vi "COPY_TEST_Approach-Retraction-VI-NanoHS50-Host-with-averager-2013-04-23-1a-data-storage-no-real-time-display.vi"() -> ()   [LabVIEW 2012]
uses:
  <vilib>/rvi/interface/nirviOpenFPGA/nirviOpenFPGA.xnode
  <vilib>/rvi/interface/nirviReadWriteControl/nirviReadWriteControl.xnode
  <vilib>/rvi/interface/nirviCloseFPGA/nirviCloseFPGA.xnode
  <vilib>/rvi/interface/nirviMethod/nirviMethod.xnode
  <vilib>/rvi/errors/niLvFpgaMergeErrorWithErrorCode.vi
  <vilib>/Utility/file.llb/Write To Spreadsheet File (I64).vi
  <vilib>/FPGAPlugInAG/PCI-7831R/niLvFpga_Open_PCI-7831R.vi
  NiFpgaLv.dll
  <vilib>/Utility/error.llb/Error Cluster From Error Code.vi
  <vilib>/rvi/errors/niLvFpgaAdjustHostInterfaceError.vi
  <vilib>/FPGAPlugInAG/PCI-7831R/niLvFpga_ReadFifo_PCI-7831R.vi
  <vilib>/FPGAPlugInAG/PCI-7831R/niLvFpga_Close_PCI-7831R.vi
  Documents/FPGA-project-apporach-retraction/FPGA Bitfiles/Apporach-Retract_FPGATarget_Automatic-Approa_WyO6UgcJbxk.lvbitx
  Downloads/labview/Automatic-Approach-Retraction-MCL-2013-04-28-1a-data-storage-1b.vi
  <vilib>/FPGAPlugInAG/PCI-7831R/niLvFpga_Run_PCI-7831R.vi
  <vilib>/FPGAPlugInAG/PCI-7831R/niLvFpga_Abort_PCI-7831R.vi
panel:
  out "Base-file-name":string="approach-15a1"
  out "Final file name":path=path "C:/Users/Rodolfo/Documents/LAB/2013-05-16-SPM-data/approach-15a1.txt"
  in  "Data Acquisition\nRate (usec)":u32=2000
  in  "start acquisition - non curve":bool
  in  "base path":path=path "C:/Users/Rodolfo/Documents/LAB/2013-05-16-SPM-data"
  in  "name-file":string="approach-15a"
  out "Data storage":bool
  in  "10 nm step":i16
  in  "variable steps":bool
  out "x*y 2":dbl=125.0
  out "x*y":dbl=3333.3333333333276
  in  "Safetip Control ON/Off":bool
  in  "safetip time wait":u32=65534
  in  "Safetip retraction":u16=1
  out "AI2-data2file":i16[](array[numeric])=[-198, -198, -198, -198, -198, -198, -198, -198, -198, -198, -197, -197, -197, -197, -197, -197, -197, -197, -197, -197, -197, -197, -197, -197, -197, -197, -196, -197, -196, -196, -196, -196, -196, -196, -196, -196, -196, -196, -196, -196, -196, -196, -196, -196, -196, -196, -196, -195, -195, -195, -195, -195, -195, -195, -195, -195, -195, -195, -195, -195, -195, -195, -195, -195, -195, -194, -194, -194, -194, -194, -194, -194, -194, -194, -194, -194, -194, -194, -194, -194, -194, -194, -194, -193, -193, -193, -193, -193, -193, -193, -193, -193, -193, -193, -193, -193, -193, -193, -193, -193, -193, -193, -193, -193, -193, -192, -192, -192, -192, -192, -192, -192, -192, -192, -192, -192, -192, -192, -192, -192, -192, -192, -191, -191, -191, -191, -191, -191, -191, -191, -191, -191, -191, -191, -191, -191, -191, -191, -191, -191, -191, -191, -190, -190, -190, -190, -190, -190, -190, -190, -190, -190, -190, -190, -190, -190, -190, -190, -190, -190, -189, -189, -189, -189, -189, -189, -189, -189, -189, -189, -189, -189, -189, -189, -189, -189, -189, -189, -188, -188, -188, -188, -188, -188, -188, -188, -188, -188, -188, -188, -188, -188, -188, -188, -188, -188, -188, -188, -187, -188, -187, -187, -187, -187, -187, -187, -187, -187, -187, -187, -187, -187, -187, -187, -187, -187, -186, -186, -186, -186, -186, -186, -186, -186, -186, -186, -186, -186, -186, -186, -186, -186, -186, -186, -186, -186, -186, -185, -185, -185, -185, -185, -185, -185, -185, -185, -185, -185, -185, -185, -185, -185, -185, -185, -185, -184, -184, -184, -184, -184, -184, -184, -184, -184, -184, -184, -184, -184, -184, -184, -184, -184, -184, -183, -184, -183, -183, -183, -183, -183, -183, -183, -183, -183, -183, -183, -183, -183, -183, -183, -183, -182, -182, -182, -182, -182, -182, -182, -182, -182, -182, -182, -182, -182, -182, -182, -182, -182, -182, -182, -182, -182, -181, -181, -181, -181, -181, -181, -181, -181, -181, -181, -181, -181, -181, -181, -181, -181, -181, -180, -180, -180, -180, -180, -180, -180, -180, -180, -180, -180, -180, -180, -180, -180, -180, -180, -180, -180, -179, -179, -180, -179, -179, -179, -179, -179, -179, -179, -179, -179, -179, -179, -179, -179, -179, -179, -179, -178, -178, -178, -178, -178, -178, -178, -178, -178, -178, -178, -178, -178, -178, -178, -178, -178, -178, -178, -177, -178, -177, -177, -177, -177, -177, -177, -177, -177, -177, -177, -177, -177, -177, -177, -177, -177, -177, -177, -176, -176, -176, -176, -176, -176, -176, -176, -176, -176, -176, -176, -176, -176, -176, -176, -175, -175, -175, -175, -175, -175, -175, -175, -175, -175, -175, -175, -175, -175, -175, -175, -175, -175, -175, -175, -175, -175, -174, -174, -174, -174, -174, -174, -174, -174, -174, -174, -174, -174, -174, -174, -174, -174, -174, -173, -174, -173, -173, -173, -173, -173, -173, -173, -173, -173, -173, -173, -173, -173, -173, -173, -173, -173, -173, -172, -172, -172, -172, -172, -172, -172, -172, -172, -172, -172, -172, -172, -172, -172, -172, -172, -171, -171]
  out "AI5-data2file":i16[](array[numeric])=[286, 288, 287, 294, 295, 295, 294, 294, 301, 300, 301, 299, 299, 297, 297, 297, 297, 297, 304, 304, 305, 307, 307, 306, 306, 308, 315, 314, 310, 311, 310, 310, 310, 310, 310, 310, 309, 309, 311, 311, 309, 307, 307, 304, 304, 301, 297, 297, 286, 286, 284, 281, 282, 271, 272, 267, 260, 260, 251, 251, 248, 244, 244, 238, 238, 235, 231, 232, 226, 226, 221, 214, 215, 201, 202, 197, 192, 192, 181, 183, 181, 180, 180, 169, 170, 169, 168, 168, 163, 163, 164, 167, 167, 167, 167, 167, 167, 167, 168, 168, 168, 169, 169, 172, 172, 176, 180, 180, 190, 189, 192, 195, 195, 210, 208, 214, 219, 218, 233, 231, 238, 242, 242, 254, 253, 262, 269, 268, 278, 277, 283, 288, 288, 302, 300, 308, 313, 313, 325, 323, 327, 329, 329, 338, 336, 343, 347, 347, 356, 354, 360, 362, 362, 365, 365, 365, 366, 366, 366, 366, 363, 361, 360, 352, 353, 350, 349, 349, 340, 341, 335, 333, 332, 321, 322, 321, 320, 320, 316, 316, 315, 314, 314, 310, 311, 305, 303, 303, 300, 301, 300, 299, 299, 297, 297, 292, 291, 290, 282, 282, 279, 278, 277, 273, 273, 274, 274, 274, 274, 274, 273, 273, 273, 274, 274, 276, 276, 277, 282, 281, 284, 284, 284, 286, 286, 287, 287, 287, 286, 286, 284, 284, 284, 281, 282, 278, 277, 276, 271, 272, 267, 267, 266, 264, 264, 261, 261, 260, 256, 257, 258, 258, 257, 253, 253, 249, 249, 247, 241, 242, 232, 231, 229, 221, 222, 212, 211, 210, 205, 205, 200, 199, 198, 190, 191, 183, 183, 182, 178, 179, 180, 180, 180, 180, 180, 182, 181, 181, 180, 180, 184, 185, 186, 190, 190, 190, 190, 190, 191, 191, 190, 190, 190, 191, 190, 195, 196, 199, 210, 209, 221, 221, 225, 237, 235, 247, 247, 251, 262, 261, 272, 271, 275, 280, 280, 294, 294, 296, 299, 299, 307, 307, 309, 315, 314, 319, 319, 320, 324, 324, 328, 328, 331, 337, 337, 343, 343, 345, 349, 349, 360, 360, 362, 365, 364, 370, 369, 369, 369, 369, 365, 365, 365, 366, 366, 361, 361, 361, 360, 360, 360, 360, 360, 358, 358, 360, 360, 359, 358, 359, 356, 356, 353, 350, 350, 346, 345, 346, 347, 347, 341, 342, 341, 340, 340, 333, 333, 333, 331, 332, 327, 327, 325, 322, 322, 320, 320, 320, 320, 320, 317, 317, 318, 320, 320, 318, 319, 321, 324, 324, 324, 324, 326, 326, 326, 330, 329, 333, 336, 336, 348, 346, 352, 357, 356, 362, 361, 364, 366, 366, 368, 368, 371, 373, 373, 373, 373, 371, 368, 368, 370, 369, 371, 372, 372, 373, 373, 373, 373, 373, 375, 374, 375, 375, 375, 367, 368, 366, 366, 365, 359, 360, 357, 355, 355, 350, 350, 344, 342, 341, 336, 337, 330, 327, 326, 319, 319, 313, 310, 310, 305, 305, 302, 301, 300, 297, 297, 297, 296, 296]
  out "Top-data2file":i32[](array[numeric])=[6625035, 6625035, 6625035, 6625035, 6625035, 6625035, 6625035, 6625035, 6625035, 6625035, 6625035, 6625035, 6625035, 6625035, 6625035, 6625035, 6625035, 6625035, 6625035, 6625035, 6625035, 6625035, 6625035, 6625035, 6625035, 6625035, 6625035, 6625035, 6625035, 6625035, 6625035, 6625035, 6625035, 6625035, 6625035, 6625035, 6625035, 6625035, 6625035, 6625035, 6625035, 6625035, 6625035, 6625035, 6625035, 6625035, 6625035, 6625035, 6625035, 6625035, 6625035, 6625035, 6625035, 6625035, 6625035, 6625035, 6625035, 6625035, 6625035, 6625035, 6625035, 6625035, 6625035, 6625035, 6625035, 6625035, 6625035, 6625035, 6625035, 6625035, 6625035, 6625035, 6625035, 6625035, 6625035, 6625035, 6625035, 6625035, 6625035, 6625035, 6625035, 6625035, 6625035, 6625035, 6625035, 6625035, 6625035, 6625035, 6625035, 6625035, 6625035, 6625035, 6625035, 6625035, 6625035, 6625035, 6625035, 6625035, 6625035, 6625035, 6625035, 6625035, 6625035, 6625035, 6625035, 6625035, 6625035, 6625035, 6625035, 6625035, 6625035, 6625035, 6625035, 6625035, 6625035, 6625035, 6625035, 6625035, 6625035, 6625035, 6625035, 6625035, 6625035, 6625035, 6625035, 6625035, 6625035, 6625035, 6625035, 6625035, 6625035, 6625035, 6625035, 6625035, 6625035, 6625035, 6625035, 6625035, 6625035, 6625035, 6625035, 6625035, 6625035, 6625035, 6625035, 6625035, 6625035, 6625035, 6625035, 6625035, 6625035, 6625035, 6625035, 6625035, 6625035, 6625035, 6625035, 6625035, 6625035, 6625035, 6625035, 6625035, 6625035, 6625035, 6625035, 6625035, 6625035, 6625035, 6625035, 6625035, 6625035, 6625035, 6625035, 6625035, 6625035, 6625035, 6625035, 6625035, 6625035, 6625035, 6625035, 6625035, 6625035, 6625035, 6625035, 6625035, 6625035, 6625035, 6625035, 6625035, 6625035, 6625035, 6625035, 6625035, 6625035, 6625035, 6625035, 6625035, 6625035, 6625035, 6625035, 6625035, 6625035, 6625035, 6625035, 6625035, 6625035, 6625035, 6625035, 6625035, 6625035, 6625035, 6625035, 6625035, 6625035, 6625035, 6625035, 6625035, 6625035, 6625035, 6625035, 6625035, 6625035, 6625035, 6625035, 6625035, 6625035, 6625035, 6625035, 6625035, 6625035, 6625035, 6625035, 6625035, 6625035, 6625035, 6625035, 6625035, 6625035, 6625035, 6625035, 6625035, 6625035, 6625035, 6625035, 6625035, 6625035, 6625035, 6625035, 6625035, 6625035, 6625035, 6625035, 6625035, 6625035, 6625035, 6625035, 6625035, 6625035, 6625035, 6625035, 6625035, 6625035, 6625035, 6625035, 6625035, 6625035, 6625035, 6625035, 6625035, 6625035, 6625035, 6625035, 6625035, 6625035, 6625035, 6625035, 6625035, 6625035, 6625035, 6625035, 6625035, 6625035, 6625035, 6625035, 6625035, 6625035, 6625035, 6625035, 6625035, 6625035, 6625035, 6625035, 6625035, 6625035, 6625035, 6625035, 6625035, 6625035, 6625035, 6625035, 6625035, 6625035, 6625035, 6625035, 6625035, 6625035, 6625035, 6625035, 6625035, 6625035, 6625035, 6625035, 6625035, 6625035, 6625035, 6625035, 6625035, 6625035, 6625035, 6625035, 6625035, 6625035, 6625035, 6625035, 6625035, 6625035, 6625035, 6625035, 6625035, 6625035, 6625035, 6625035, 6625035, 6625035, 6625035, 6625035, 6625035, 6625035, 6625035, 6625035, 6625035, 6625035, 6625035, 6625035, 6625035, 6625035, 6625035, 6625035, 6625035, 6625035, 6625035, 6625035, 6625035, 6625035, 6625035, 6625035, 6625035, 6625035, 6625035, 6625035, 6625035, 6625035, 6625035, 6625035, 6625035, 6625035, 6625035, 6625035, 6625035, 6625035, 6625035, 6625035, 6625035, 6625035, 6625035, 6625035, 6625035, 6625035, 6625035, 6625035, 6625035, 6625035, 6625035, 6625035, 6625035, 6625035, 6625035, 6625035, 6625035, 6625035, 6625035, 6625035, 6625035, 6625035, 6625035, 6625035, 6625035, 6625035, 6625035, 6625035, 6625035, 6625035, 6625035, 6625035, 6625035, 6625035, 6625035, 6625035, 6625035, 6625035, 6625035, 6625035, 6625035, 6625035, 6625035, 6625035, 6625035, 6625035, 6625035, 6625035, 6625035, 6625035, 6625035, 6625035, 6625035, 6625035, 6625035, 6625035, 6625035, 6625035, 6625035, 6625035, 6625035, 6625035, 6625035, 6625035, 6625035, 6625035, 6625035, 6625035, 6625035, 6625035, 6625035, 6625035, 6625035, 6625035, 6625035, 6625035, 6625035, 6625035, 6625035, 6625035, 6625035, 6625035, 6625035, 6625035, 6625035, 6625035, 6625035, 6625035, 6625035, 6625035, 6625035, 6625035, 6625035, 6625035, 6625035, 6625035, 6625035, 6625035, 6625035, 6625035, 6625035, 6625035, 6625035, 6625035, 6625035, 6625035, 6625035, 6625035, 6625035, 6625035, 6625035, 6625035, 6625035, 6625035, 6625035, 6625035, 6625035, 6625035, 6625035, 6625035, 6625035, 6625035, 6625035, 6625035, 6625035, 6625035, 6625035]
  out "AI6-data2file":i16[](array[numeric])=[10327, 10323, 10323, 10324, 10324, 10324, 10323, 10323, 10321, 10320, 10320, 10318, 10318, 10312, 10310, 10309, 10304, 10305, 10298, 10296, 10296, 10301, 10301, 10298, 10297, 10297, 10290, 10290, 10294, 10295, 10295, 10296, 10296, 10303, 10304, 10305, 10309, 10308, 10308, 10307, 10307, 10309, 10308, 10309, 10309, 10310, 10319, 10318, 10318, 10318, 10318, 10317, 10317, 10310, 10308, 10308, 10307, 10307, 10308, 10308, 10308, 10304, 10304, 10298, 10296, 10295, 10291, 10291, 10287, 10286, 10286, 10285, 10285, 10290, 10291, 10292, 10294, 10294, 10295, 10295, 10295, 10294, 10294, 10297, 10297, 10298, 10301, 10301, 10307, 10307, 10308, 10311, 10311, 10310, 10309, 10311, 10319, 10318, 10320, 10320, 10320, 10319, 10319, 10320, 10320, 10320, 10319, 10319, 10318, 10318, 10317, 10314, 10314, 10308, 10307, 10307, 10304, 10304, 10307, 10307, 10307, 10308, 10308, 10310, 10311, 10312, 10314, 10314, 10314, 10314, 10315, 10317, 10317, 10318, 10318, 10318, 10318, 10318, 10314, 10313, 10313, 10311, 10311, 10307, 10307, 10307, 10309, 10308, 10308, 10308, 10308, 10308, 10308, 10308, 10308, 10307, 10303, 10303, 10301, 10301, 10301, 10301, 10301, 10304, 10303, 10305, 10309, 10308, 10310, 10309, 10313, 10321, 10320, 10324, 10324, 10329, 10337, 10336, 10341, 10341, 10341, 10342, 10342, 10341, 10341, 10337, 10331, 10331, 10317, 10317, 10314, 10310, 10311, 10303, 10303, 10300, 10294, 10295, 10287, 10288, 10288, 10287, 10287, 10285, 10285, 10286, 10286, 10286, 10295, 10295, 10297, 10301, 10301, 10311, 10310, 10314, 10318, 10318, 10319, 10319, 10323, 10328, 10328, 10334, 10333, 10335, 10337, 10337, 10337, 10337, 10337, 10336, 10336, 10331, 10331, 10329, 10327, 10327, 10324, 10324, 10322, 10320, 10320, 10313, 10313, 10314, 10314, 10314, 10308, 10308, 10306, 10304, 10304, 10309, 10308, 10303, 10299, 10300, 10301, 10301, 10302, 10305, 10304, 10300, 10301, 10303, 10305, 10304, 10303, 10303, 10304, 10305, 10305, 10308, 10308, 10308, 10308, 10308, 10315, 10314, 10316, 10317, 10317, 10321, 10320, 10324, 10328, 10328, 10334, 10333, 10336, 10337, 10337, 10340, 10339, 10342, 10343, 10343, 10343, 10343, 10346, 10347, 10347, 10347, 10347, 10349, 10349, 10349, 10347, 10347, 10344, 10343, 10343, 10343, 10343, 10343, 10343, 10343, 10339, 10340, 10338, 10337, 10337, 10333, 10334, 10327, 10324, 10324, 10320, 10320, 10318, 10317, 10316, 10310, 10311, 10300, 10297, 10296, 10284, 10286, 10285, 10285, 10285, 10284, 10284, 10287, 10288, 10289, 10298, 10297, 10303, 10304, 10306, 10319, 10317, 10330, 10332, 10334, 10348, 10347, 10349, 10350, 10350, 10355, 10354, 10354, 10354, 10354, 10349, 10349, 10344, 10343, 10342, 10332, 10334, 10326, 10324, 10323, 10313, 10315, 10310, 10310, 10309, 10308, 10308, 10304, 10304, 10302, 10294, 10295, 10292, 10291, 10290, 10286, 10287, 10285, 10285, 10285, 10281, 10281, 10285, 10285, 10286, 10288, 10288, 10290, 10290, 10291, 10295, 10295, 10299, 10300, 10302, 10312, 10311, 10320, 10320, 10321, 10323, 10323, 10320, 10320, 10321, 10324, 10323, 10324, 10324, 10325, 10328, 10327, 10327, 10326, 10328, 10332, 10331, 10330, 10330, 10332, 10338, 10337, 10341, 10341, 10340, 10336, 10336, 10334, 10333, 10333, 10330, 10331, 10331, 10331, 10330, 10327, 10328, 10330, 10330, 10328, 10323, 10324, 10317, 10317, 10316, 10314, 10315, 10314, 10314, 10312, 10307, 10307, 10301, 10301, 10297, 10290, 10291, 10285, 10285, 10283, 10277, 10278, 10277, 10277, 10279, 10282, 10282, 10286, 10286, 10288, 10292, 10291, 10301, 10300, 10304, 10308, 10307, 10318, 10318, 10320, 10324, 10323]
  out "AI1-data2file":i16[](array[numeric])
  out "AI7-data2file":i16[](array[numeric])=[26628, 26626, 26633, 26632, 26632, 26626, 26648, 26626, 26639, 26625, 26644, 26635, 26624, 26639, 26643, 26622, 26621, 26637, 26626, 26627, 26641, 26632, 26634, 26652, 26632, 26635, 26620, 26631, 26645, 26637, 26634, 26631, 26640, 26634, 26640, 26632, 26637, 26642, 26623, 26629, 26624, 26638, 26636, 26646, 26622, 26644, 26622, 26624, 26636, 26632, 26636, 26617, 26628, 26639, 26639, 26626, 26628, 26650, 26634, 26626, 26641, 26620, 26628, 26639, 26625, 26646, 26618, 26649, 26627, 26641, 26625, 26638, 26636, 26636, 26638, 26639, 26638, 26640, 26642, 26641, 26639, 26628, 26638, 26629, 26639, 26631, 26638, 26638, 26625, 26636, 26635, 26628, 26652, 26635, 26632, 26628, 26644, 26632, 26644, 26638, 26633, 26616, 26630, 26629, 26623, 26630, 26623, 26633, 26626, 26644, 26636, 26643, 26625, 26632, 26632, 26633, 26630, 26623, 26623, 26636, 26632, 26631, 26637, 26632, 26633, 26640, 26646, 26632, 26635, 26629, 26635, 26621, 26633, 26634, 26628, 26642, 26634, 26629, 26619, 26639, 26632, 26632, 26636, 26634, 26637, 26633, 26644, 26631, 26647, 26626, 26646, 26628, 26633, 26642, 26653, 26640, 26633, 26638, 26633, 26620, 26641, 26640, 26630, 26621, 26621, 26644, 26642, 26634, 26641, 26627, 26615, 26640, 26633, 26639, 26628, 26634, 26647, 26623, 26625, 26635, 26639, 26640, 26629, 26640, 26614, 26656, 26630, 26649, 26652, 26630, 26637, 26620, 26638, 26632, 26638, 26646, 26633, 26628, 26645, 26636, 26639, 26632, 26633, 26649, 26627, 26633, 26629, 26631, 26629, 26643, 26627, 26631, 26637, 26635, 26648, 26629, 26635, 26636, 26640, 26627, 26640, 26608, 26640, 26629, 26632, 26646, 26632, 26629, 26631, 26621, 26643, 26640, 26618, 26623, 26640, 26640, 26639, 26628, 26630, 26636, 26631, 26642, 26633, 26639, 26633, 26647, 26624, 26630, 26631, 26646, 26630, 26636, 26638, 26636, 26647, 26638, 26625, 26625, 26631, 26625, 26639, 26638, 26641, 26625, 26650, 26634, 26643, 26607, 26660, 26623, 26642, 26649, 26631, 26633, 26632, 26641, 26627, 26632, 26641, 26627, 26646, 26629, 26618, 26635, 26630, 26643, 26627, 26639, 26630, 26625, 26625, 26639, 26641, 26626, 26638, 26630, 26628, 26649, 26637, 26632, 26625, 26630, 26641, 26638, 26636, 26632, 26627, 26628, 26629, 26642, 26631, 26619, 26636, 26628, 26631, 26634, 26633, 26640, 26627, 26645, 26628, 26633, 26625, 26637, 26617, 26628, 26637, 26642, 26628, 26643, 26637, 26637, 26629, 26632, 26629, 26633, 26626, 26637, 26630, 26635, 26637, 26653, 26634, 26636, 26638, 26623, 26629, 26638, 26630, 26638, 26649, 26622, 26640, 26635, 26629, 26627, 26651, 26643, 26652, 26625, 26631, 26627, 26637, 26631, 26626, 26630, 26627, 26646, 26629, 26644, 26632, 26652, 26636, 26628, 26644, 26651, 26623, 26639, 26622, 26643, 26635, 26661, 26635, 26630, 26631, 26638, 26631, 26632, 26629, 26625, 26629, 26627, 26622, 26636, 26637, 26628, 26638, 26631, 26625, 26627, 26630, 26639, 26646, 26629, 26631, 26650, 26620, 26634, 26634, 26652, 26626, 26644, 26639, 26639, 26646, 26646, 26631, 26640, 26630, 26638, 26638, 26651, 26633, 26631, 26622, 26641, 26639, 26639, 26637, 26633, 26630, 26647, 26619, 26640, 26641, 26630, 26642, 26633, 26629, 26641, 26623, 26631, 26647, 26618, 26641, 26630, 26638, 26631, 26634, 26631, 26633, 26637, 26631, 26635, 26635, 26637, 26640, 26636, 26631, 26634, 26644, 26632, 26642, 26630, 26626, 26629, 26641, 26641, 26636, 26640, 26639, 26639, 26629, 26640, 26629, 26647, 26625, 26647, 26651, 26636, 26633, 26625, 26629, 26638, 26644, 26639, 26602, 26636, 26621, 26629, 26636, 26643, 26633, 26640, 26632, 26631, 26633, 26636, 26624, 26627]
  out "AI4-data2file":i16[](array[numeric])=[355, 354, 354, 355, 355, 354, 353, 352, 351, 350, 351, 351, 350, 349, 350, 350, 350, 351, 352, 353, 353, 353, 352, 350, 349, 346, 345, 345, 342, 340, 339, 341, 342, 342, 344, 345, 345, 346, 348, 348, 347, 348, 348, 347, 346, 346, 345, 346, 344, 345, 347, 348, 349, 350, 350, 352, 353, 353, 353, 352, 351, 350, 350, 352, 353, 353, 355, 354, 353, 353, 355, 353, 355, 354, 355, 356, 356, 356, 354, 352, 352, 350, 350, 350, 350, 350, 350, 350, 350, 348, 347, 345, 346, 346, 346, 346, 346, 346, 345, 344, 346, 346, 347, 347, 349, 349, 347, 347, 346, 348, 349, 349, 349, 349, 349, 349, 349, 348, 351, 350, 350, 352, 354, 355, 354, 353, 351, 350, 349, 347, 348, 347, 347, 345, 345, 345, 345, 345, 345, 345, 347, 346, 346, 345, 345, 344, 346, 346, 346, 347, 348, 351, 350, 350, 350, 350, 352, 352, 352, 350, 350, 350, 350, 350, 350, 351, 351, 350, 350, 349, 348, 347, 345, 345, 347, 349, 349, 349, 349, 349, 350, 350, 352, 352, 351, 349, 346, 346, 345, 343, 342, 340, 341, 341, 341, 340, 340, 341, 340, 340, 341, 343, 345, 345, 348, 349, 349, 350, 350, 351, 351, 350, 350, 350, 351, 351, 351, 350, 350, 352, 353, 353, 353, 355, 355, 355, 355, 355, 353, 352, 352, 352, 352, 353, 353, 355, 355, 354, 355, 355, 355, 355, 355, 353, 353, 351, 350, 350, 350, 350, 351, 350, 350, 350, 350, 350, 351, 351, 352, 353, 353, 353, 353, 353, 355, 356, 356, 357, 359, 359, 359, 359, 359, 359, 359, 359, 359, 358, 359, 359, 359, 359, 359, 359, 357, 358, 357, 356, 354, 353, 352, 351, 350, 349, 349, 348, 347, 347, 345, 344, 345, 345, 345, 344, 345, 346, 347, 348, 351, 350, 350, 353, 353, 353, 353, 353, 352, 350, 351, 350, 347, 346, 345, 346, 346, 346, 347, 349, 350, 352, 353, 352, 351, 351, 351, 351, 350, 350, 350, 349, 349, 349, 349, 348, 348, 346, 346, 346, 346, 346, 349, 349, 351, 350, 350, 352, 355, 354, 355, 355, 354, 351, 350, 350, 351, 352, 352, 354, 355, 355, 354, 353, 352, 350, 350, 350, 348, 347, 345, 344, 344, 343, 344, 342, 342, 342, 343, 344, 345, 349, 350, 352, 355, 356, 356, 356, 356, 355, 354, 352, 353, 350, 351, 350, 350, 349, 349, 349, 349, 348, 346, 346, 346, 345, 345, 345, 344, 343, 343, 344, 345, 344, 345, 344, 345, 345, 345, 345, 345, 343, 342, 342, 340, 342, 340, 341, 341, 343, 343, 345, 344, 345, 345, 345, 345, 344, 345, 345, 345, 345, 347, 348, 348, 349, 349, 349, 348, 347, 346, 345, 345, 344, 343, 343, 342, 342, 343, 343, 345, 345, 345, 345, 346, 347, 349, 349, 351, 350, 350, 350, 350, 350, 350, 349, 349, 349, 348, 347, 346, 345, 345, 346, 347, 347, 346, 345, 345, 345, 345, 345]
  in  "start acquisition":bool
  out "Phase 1":bool
  in  "phase 1 control":bool
  out "Initial Height (Fine)":i16
  out "MCL counter in range?":bool=TRUE
  out "Zposition MCL fine":i16=6000
  out "MCL counter":u16=101
  out "Curve indicator":u16=1
  in  "Manual Control":bool=TRUE
  in  "Start Approach":bool
  in  "Data Length":i32=10000
  in  "MCL  Divisions":u16=102
  in  "MCL counter 2":u16=101
  in  "Zposition MCL fine 2":i16=6000 step=1
  in  "Initial Position":i16
  in  "Safetip Minimum":i16=4700
  in  "Number of curves":u16=5
  in  "Fine Retraction  Velocity (nm/s)":dbl=3.0000000000000053 format="%.2g"
  in  "Wait-tip-before-new-approach (usec)":u32=100000
  in  "Wait-tip-\nbefore-approach (usec)":u32=100001
  in  "Fast Approach\nVelocity (nm/s)":dbl=80.0 min=0.1 max=100.0 step=0.001 format="%_3g"
  in  "Approach Setpoint":i16=16400
  out "Signal away from surface":i16=26655
  in  "First fast\napproach offset":i16=90
  in  "Fast Retraction\nbefore approach":i32=3601 min=0
  in  "Minimum for Approach Value":i16=7800
  in  "Fast Retraction after approach":i32=30000 step=1
  out "AI2":i16[](graph)
  out "AI5":i16[](graph)
  out "Topography":i32[](graph)
  out "AI6":i16[](graph)
  out "AI1":i16[](graph)
  out "AI7":i16[](graph)
  out "AI4":i16[](graph)
  out "Data 2":u64[](array[numeric])=[28454742470360890, 28454742470491962, 28454742470426426, 28454742470885178, 28454742470950714, 28454742470950714, 28454742470885178, 28454742470885178, 28454742471343930, 28454742471278394, 28454742471343931, 28454742471212859, 28454742471212859, 28454742471081787, 28454742471081787, 28454742471081787, 28454742471081787, 28454742471081787, 28454742471540539, 28454742471540539, 28454742471606075, 28454742471737147, 28454742471737147, 28454742471671611, 28454742471671611, 28454742471802683, 28454742472261436, 28454742472195899, 28454742471933756, 28454742471999292, 28454742471933756, 28454742471933756, 28454742471933756, 28454742471933756, 28454742471933756, 28454742471933756, 28454742471868220, 28454742471868220, 28454742471999292, 28454742471999292, 28454742471868220, 28454742471737148, 28454742471737148, 28454742471540540, 28454742471540540, 28454742471343932, 28454742471081788, 28454742471081789, 28454742470360893, 28454742470360893, 28454742470229821, 28454742470033213, 28454742470098749, 28454742469377853, 28454742469443389, 28454742469115709, 28454742468656957, 28454742468656957, 28454742468067133, 28454742468067133, 28454742467870525, 28454742467608381, 28454742467608381, 28454742467215165, 28454742467215165, 28454742467018558, 28454742466756414, 28454742466821950, 28454742466428734, 28454742466428734, 28454742466101054, 28454742465642302, 28454742465707838, 28454742464790334, 28454742464855870, 28454742464528190, 28454742464200510, 28454742464200510, 28454742463479614, 28454742463610686, 28454742463479614, 28454742463414078, 28454742463414078, 28454742462693183, 28454742462758719, 28454742462693183, 28454742462627647, 28454742462627647, 28454742462299967, 28454742462299967, 28454742462365503, 28454742462562111, 28454742462562111, 28454742462562111, 28454742462562111, 28454742462562111, 28454742462562111, 28454742462562111, 28454742462627647, 28454742462627647, 28454742462627647, 28454742462693183, 28454742462693183, 28454742462889791, 28454742462889791, 28454742463151936, 28454742463414080, 28454742463414080, 28454742464069440, 28454742464003904, 28454742464200512, 28454742464397120, 28454742464397120, 28454742465380160, 28454742465249088, 28454742465642304, 28454742465969984, 28454742465904448, 28454742466887488, 28454742466756416, 28454742467215168, 28454742467477312, 28454742467477313, 28454742468263745, 28454742468198209, 28454742468788033, 28454742469246785, 28454742469181249, 28454742469836609, 28454742469771073, 28454742470164289, 28454742470491969, 28454742470491969, 28454742471409473, 28454742471278401, 28454742471802689, 28454742472130369, 28454742472130369, 28454742472916801, 28454742472785729, 28454742473047873, 28454742473178945, 28454742473178946, 28454742473768770, 28454742473637698, 28454742474096450, 28454742474358594, 28454742474358594, 28454742474948418, 28454742474817346, 28454742475210562, 28454742475341634, 28454742475341634, 28454742475538242, 28454742475538242, 28454742475538242, 28454742475603778, 28454742475603778, 28454742475603778, 28454742475603778, 28454742475407171, 28454742475276099, 28454742475210563, 28454742474686275, 28454742474751811, 28454742474555203, 28454742474489667, 28454742474489667, 28454742473899843, 28454742473965379, 28454742473572163, 28454742473441091, 28454742473375555, 28454742472654659, 28454742472720195, 28454742472654659, 28454742472589123, 28454742472589123, 28454742472326980, 28454742472326980, 28454742472261444, 28454742472195908, 28454742472195908, 28454742471933764, 28454742471999300, 28454742471606084, 28454742471475012, 28454742471475012, 28454742471278404, 28454742471343940, 28454742471278404, 28454742471212868, 28454742471212868, 28454742471081796, 28454742471081796, 28454742470754116, 28454742470688580, 28454742470623044, 28454742470098757, 28454742470098756, 28454742469902149, 28454742469836613, 28454742469771077, 28454742469508933, 28454742469508933, 28454742469574469, 28454742469574469, 28454742469574469, 28454742469574469, 28454742469574469, 28454742469508933, 28454742469508933, 28454742469508933, 28454742469574469, 28454742469574469, 28454742469705541, 28454742469705542, 28454742469771078, 28454742470098758, 28454742470033222, 28454742470229830, 28454742470229830, 28454742470229830, 28454742470360902, 28454742470360902, 28454742470426438, 28454742470426438, 28454742470426438, 28454742470360902, 28454742470360902, 28454742470229830, 28454742470229830, 28454742470229830, 28454742470033222, 28454742470098758, 28454742469836614, 28454742469771078, 28454742469705543, 28454742469377863, 28454742469443399, 28454742469115719, 28454742469115719, 28454742469050183, 28454742468919111, 28454742468919111, 28454742468722503, 28454742468722503, 28454742468656967, 28454742468394823, 28454742468460359, 28454742468525895, 28454742468525895, 28454742468460359, 28454742468198215, 28454742468198215, 28454742467936072, 28454742467936072, 28454742467805000, 28454742467411784, 28454742467477320, 28454742466821960, 28454742466756424, 28454742466625352, 28454742466101064, 28454742466166600, 28454742465511240, 28454742465445704, 28454742465380168, 28454742465052488, 28454742465052488, 28454742464724808, 28454742464659272, 28454742464593736, 28454742464069449, 28454742464134984, 28454742463610697, 28454742463610697, 28454742463545161, 28454742463283017, 28454742463348553, 28454742463414089, 28454742463414089, 28454742463414089, 28454742463414089, 28454742463414089, 28454742463545161, 28454742463479625, 28454742463479625, 28454742463414089, 28454742463414089, 28454742463676233, 28454742463741770, 28454742463807306, 28454742464069450, 28454742464069450, 28454742464069450, 28454742464069450, 28454742464069450, 28454742464134986, 28454742464134986, 28454742464069450, 28454742464069450, 28454742464069450, 28454742464134986, 28454742464069450, 28454742464397130, 28454742464462666, 28454742464659274, 28454742465380170, 28454742465314634, 28454742466101066, 28454742466101066, 28454742466363211, 28454742467149643, 28454742467018571, 28454742467805003, 28454742467805003, 28454742468067147, 28454742468788043, 28454742468722507, 28454742469443403, 28454742469377867, 28454742469640011, 28454742469967691, 28454742469967691, 28454742470885195, 28454742470885195, 28454742471016267, 28454742471212875, 28454742471212876, 28454742471737164, 28454742471737164, 28454742471868236, 28454742472261452, 28454742472195916, 28454742472523596, 28454742472523596, 28454742472589132, 28454742472851276, 28454742472851276, 28454742473113420, 28454742473113420, 28454742473310028, 28454742473703244, 28454742473703244, 28454742474096460, 28454742474096460, 28454742474227532, 28454742474489677, 28454742474489677, 28454742475210572, 28454742475210573, 28454742475341645, 28454742475538253, 28454742475472717, 28454742475865933, 28454742475800397, 28454742475800397, 28454742475800397, 28454742475800397, 28454742475538253, 28454742475538253, 28454742475538253, 28454742475603789, 28454742475603789, 28454742475276109, 28454742475276109, 28454742475276110, 28454742475210574, 28454742475210574, 28454742475210574, 28454742475210574, 28454742475210574, 28454742475079502, 28454742475079502, 28454742475210574, 28454742475210574, 28454742475145038, 28454742475079502, 28454742475145038, 28454742474948430, 28454742474948430, 28454742474751822, 28454742474555214, 28454742474555214, 28454742474293070, 28454742474227535, 28454742474293070, 28454742474358607, 28454742474358607, 28454742473965391, 28454742474030927, 28454742473965391, 28454742473899855, 28454742473899855, 28454742473441103, 28454742473441103, 28454742473441103, 28454742473310031, 28454742473375567, 28454742473047887, 28454742473047887, 28454742472916815, 28454742472720207, 28454742472720207, 28454742472589135, 28454742472589136, 28454742472589136, 28454742472589136, 28454742472589136, 28454742472392528, 28454742472392528, 28454742472458064, 28454742472589136, 28454742472589136, 28454742472458064, 28454742472523600, 28454742472654672, 28454742472851280, 28454742472851280, 28454742472851280, 28454742472851280, 28454742472982353, 28454742472982353, 28454742472982353, 28454742473244497, 28454742473178961, 28454742473441105, 28454742473637713, 28454742473637713, 28454742474424145, 28454742474293073, 28454742474686289, 28454742475013969, 28454742474948433, 28454742475341649, 28454742475276113, 28454742475472721, 28454742475603793, 28454742475603793, 28454742475734865, 28454742475734865, 28454742475931473, 28454742476062545, 28454742476062546, 28454742476062546, 28454742476062546, 28454742475931474, 28454742475734866, 28454742475734866, 28454742475865938, 28454742475800402, 28454742475931474, 28454742475997010, 28454742475997010, 28454742476062546, 28454742476062546, 28454742476062546, 28454742476062546, 28454742476062546, 28454742476193618, 28454742476128083, 28454742476193618, 28454742476193619, 28454742476193619, 28454742475669331, 28454742475734867, 28454742475603795, 28454742475603795, 28454742475538259, 28454742475145043, 28454742475210579, 28454742475013971, 28454742474882899, 28454742474882899, 28454742474555219, 28454742474555219, 28454742474162003, 28454742474030931, 28454742473965395, 28454742473637715, 28454742473703252, 28454742473244500, 28454742473047892, 28454742472982356, 28454742472523604, 28454742472523604, 28454742472130388, 28454742471933780, 28454742471933780, 28454742471606100, 28454742471606100, 28454742471409492, 28454742471343956, 28454742471278420, 28454742471081812, 28454742471081812, 28454742471081812, 28454742471016277, 28454742471016277]
  out "Data":u64[](array[numeric])=[100037983121451095, 99756499554805843, 99756529619576915, 100038000301320276, 100038000301320276, 99756499554805844, 99475119067375699, 99193549601384531, 98912130459248721, 98630595352995920, 98912151934085200, 98912113279379534, 98630591058028622, 98349180505827400, 98630672662407238, 98630582468094021, 98630578173126720, 98912121869314113, 99193549601384506, 99475028873062456, 99475089002604600, 99475050347898941, 99193583961122877, 98630711317112890, 98349150441056313, 97504738395826233, 97223198994606130, 97223246239246386, 96378881438656566, 95815897125496887, 95534409263884343, 96097346332403768, 96378859963820088, 96378834194016319, 96941809917241408, 97223250534213697, 97223272009050181, 97504768460597316, 98067636809640004, 98067662579443779, 97786166127896643, 98067701234149445, 98067692644214852, 97786260617177157, 97504682561251397, 97504777050531910, 97223207584540751, 97504691151185998, 96941792737372238, 97223250534213710, 97786217667504206, 98067611039836237, 98349133261187149, 98630655482538054, 98630655482538052, 99193549601384516, 99475033168029763, 99475127657310275, 99475058937833540, 99193549601384516, 98912139049183300, 98630573878159424, 98630608237897792, 99193605435959354, 99475020283127864, 99475110477441079, 100037940171778099, 99756598339053619, 99475028873062447, 99475089002604590, 100037970236549166, 99475076117702701, 100038017481189421, 99756542504478770, 100038026071124019, 100319505342801972, 100319501047834678, 100319509637769270, 99756568274282551, 99193614025893943, 99193605435959351, 98630608237897782, 98630651187570742, 98630612532865081, 98630655482538041, 98630621122799674, 98630651187570749, 98630651187570749, 98630595352995907, 98067692644214851, 97786213372536900, 97223233354344519, 97504811410270279, 97504738395826246, 97504725510924357, 97504708331055175, 97504777050531919, 97504725510924366, 97223302073821264, 96941801327306832, 97504729805891664, 97504656791447631, 97786191897700431, 97786187602733136, 98349111786350672, 98349141851121744, 97786161832929359, 97786204782602319, 97504699741120590, 98067727003953230, 98349167620925517, 98349197685696586, 98349120376285258, 98349150441056324, 98349150441056323, 98349154736023619, 98349141851121728, 98067636809640000, 98912061739771971, 98630642597636163, 98630625417766979, 99193571076220996, 99756546799446084, 100038000301320262, 99756529619576903, 99475084707637320, 98912160524019786, 98630625417766986, 98349163325958218, 97786187602733130, 98067688349247563, 97786153242994765, 97786204782602317, 97223259124148302, 97223233354344526, 97223293483886670, 97223259124148302, 97223237649311822, 97223194699638858, 97223280598984777, 97786200487635017, 97504725510924359, 97504742690793543, 97223259124148291, 97223272009050179, 96941779852470339, 97504777050531909, 97504721215957060, 97504789935433796, 97786174717831236, 98067735593887812, 98912083214608452, 98630629712734276, 98630668367439940, 98630715612080196, 98630659777505347, 99193579666155583, 99193601140992063, 99193579666155581, 98630573878159421, 98630664072472637, 98630659777505341, 98630616827832381, 98630578173126720, 98630578173126719, 98912151934085185, 98912143344150597, 98630634007701572, 98630664072472646, 98349128966219845, 98067602449901641, 97786234847373393, 97223254829181008, 97223280598984788, 97786183307765844, 98349159030990937, 98349214865565793, 98349111786350688, 98349120376285285, 98349163325958245, 98630655482538085, 98630659777505382, 99193562486286438, 99193609730926693, 98912023085066341, 98349253520271457, 97504716920989787, 97504798525368411, 97223336433559629, 96660291990857805, 96378847078918218, 95815824111052870, 96097376397174855, 96097350627371071, 96097376397174847, 95815935780202556, 95815879945627702, 96097333447501879, 95815931485235247, 95815892830529584, 96097380692142128, 96660300580792367, 97223254829180975, 97223323548657709, 98067653989509165, 98349154736023598, 98349137556154414, 98630621122799662, 98630612532865079, 98912147639117879, 98912078919641145, 98630621122799677, 98630646892603453, 98630638302668871, 98912169113954374, 98912087509575754, 98912113279379534, 98630642597636174, 98630659777505359, 99193553896351823, 99475084707637331, 99474947268683864, 99475084707637336, 100037987416418398, 100038000301320285, 100038060430862431, 100038000301320289, 100037987416418401, 99475046052931681, 99193528126548065, 99193622615828577, 99193609730926688, 99193515241646176, 99475011693193307, 99475084707637339, 100038034661058649, 100038030366091351, 99756508144740439, 100037991711385684, 100038017481189460, 100037996006352978, 100038043250993232, 100038004596287568, 99475080412670025, 99475054642866249, 98912164818987082, 98630591058028618, 98630616827832394, 98630621122799684, 98630685547309124, 98912091804543042, 98630642597636160, 98630651187570752, 98630642597636165, 98630689842276420, 98630651187570751, 98912070329706555, 98912070329706556, 99193571076220989, 99475020283127869, 99475080412670014, 99475076117702721, 99475089002604608, 99475020283127868, 100038077610731581, 100319483867965503, 100319522522671169, 100600842880559168, 101164020467247167, 101163861553457215, 101163943157835840, 101163973222606913, 101163895913195585, 101163904503130180, 101163900208162884, 101163938862868548, 101163878733326404, 100882425231452228, 101163938862868555, 101163878733326410, 101163960337705036, 101163887323261005, 101163840078620749, 101163913093064785, 100600941664806992, 100882472476092500, 100600928779905112, 100319505342802008, 99756516734675038, 99475020283127901, 99193545306417248, 98912130459248737, 98630664072472673, 98349124671252580, 98349176210860131, 98067666874411110, 97786183307765863, 97786273502079079, 97223272009050215, 96941775557503079, 97223220469442666, 97223241944279147, 97223289188919403, 96941801327306859, 97223267714082923, 97504725510924397, 97786179012798573, 98067658284476525, 98912087509575787, 98630668367439979, 98630621122799720, 99474994513324135, 99475067527768167, 99475033168029799, 99475046052931687, 99475058937833575, 99193579666155623, 98630659777505383, 98912078919641187, 98630681252341860, 97786183307765858, 97504729805891681, 97223220469442657, 97504746985760861, 97504661086414942, 97504708331055191, 97786221962471508, 98349193390729300, 98630608237897808, 99193622615828560, 99475071822735438, 99193596846024781, 98912087509575756, 98912100394477638, 98912087509575751, 98912104689444924, 98630599647963193, 98630646892603448, 98630616827832364, 98349163325958190, 98349171915892781, 98349240635369517, 98349159030990893, 98067692644214828, 98067701234149420, 97504686856218671, 97504712626022448, 97504751280728113, 97504716920989754, 97504751280728121, 98349223455500351, 98349107491383360, 98912134754216002, 98630638302668879, 98630612532865101, 99193553896351834, 100038081905698908, 99756572569249886, 100038086200666220, 100037970236549227, 99756521029642349, 98912078919641198, 98630646892603502, 98630621122799731, 98912074624673906, 99193566781253746, 99193553896351858, 99756585454151794, 100037987416418413, 100038051840927853, 99756525324609640, 99475136247244903, 99193592551057510, 98630608237897820, 98630676957374558, 98630707022145622, 98067636809640020, 97786230552406099, 97223207584540745, 96941822802143307, 96941788442404934, 96660425134843974, 96941788442404933, 96378817014147140, 96378821309114436, 96378851373885504, 96660296285825088, 96941775557503038, 97223237649311798, 98349120376285239, 98630612532865076, 99193553896351795, 100037957351647282, 100319492457900078, 100319496752867375, 100319458098161709, 100319501047834669, 100037996006352941, 99756495259838505, 99193553896351785, 99475041757964333, 98630655482538029, 98912160524019758, 98630612532865072, 98630621122799664, 98349227750467634, 98349098901448754, 98349159030990899, 98349159030990903, 98067761363691575, 97504699741120571, 97504777050531900, 97504755575695422, 97223280598984776, 97223310663755847, 97223310663755856, 96941771262535760, 96660334940530769, 96660291990857811, 96941801327306835, 97223276304017488, 96941857161881680, 97223254829181009, 96941771262535764, 97223207584540755, 97223289188919380, 97223280598984788, 97223280598984789, 97223272009050200, 96660304875759703, 96378817014147159, 96378890028591190, 95815819816085592, 96378859963820124, 95815914305366107, 96097342037436506, 96097393577044058, 96660304875759708, 96660287695890530, 97223289188919393, 96941736902797413, 97223246239246437, 97223314958723172, 97223190404671584, 97223289188919392, 96941766967568478, 97223276304017501, 97223246239246429, 97223259124148314, 97223246239246427, 97786204782602331, 98067696939182171, 98067671169378394, 98349163325958231, 98349163325958232, 98349171915892826, 98067709824084058, 97786217667504216, 97504721215957075, 97223259124148308, 97223302073821261, 96941775557503053, 96660343530465356, 96660291990857802, 96378799834277963, 96378812719179850, 96660339235498058, 96660339235498056, 97223267714082883, 97223284893952067, 97223280598984765, 97223280598984765, 97504712626022457, 97786234847373362, 98349137556154419, 98349214865565741, 98912070329706541, 98630689842276395, 98630707022145573, 98630642597636134, 98630629712734245, 98630595352995877, 98630612532865063, 98349176210860074, 98349201980663850, 98349180505827374, 98067546615326766, 97786217667504176, 97504678266284084, 97223237649311795, 97223267714082877, 97504772755564604, 97786204782602304, 97786234847373380, 97504725510924355, 97223246239246414, 97223254829181006, 97223267714082896, 97223216174475348, 97223229059377235]
  in  "Fine Approach\nVelocity (nm/s)":dbl=3.0000000000000053 min=0.001 step=0.001 format="%.2g"
  in  "Number of Elements":u32=500
  # "Freq shift"
  # "Top sensor"
  # "USBS Amp"
  # "Tunneling current"
  # "Control Signal (Aux 1)"
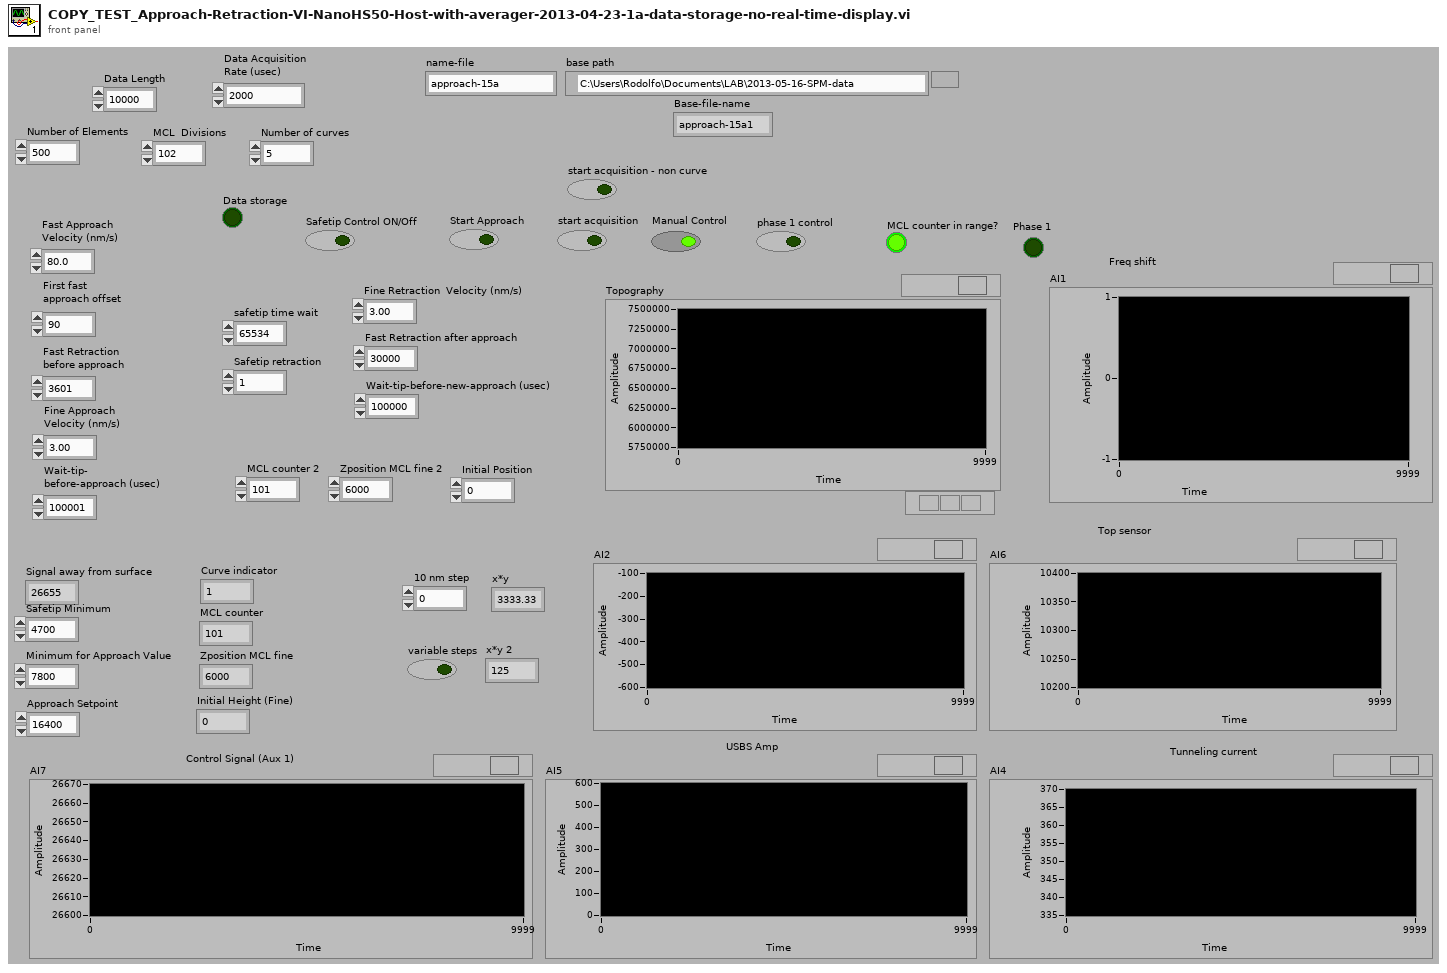
[diagram p1: front panel]
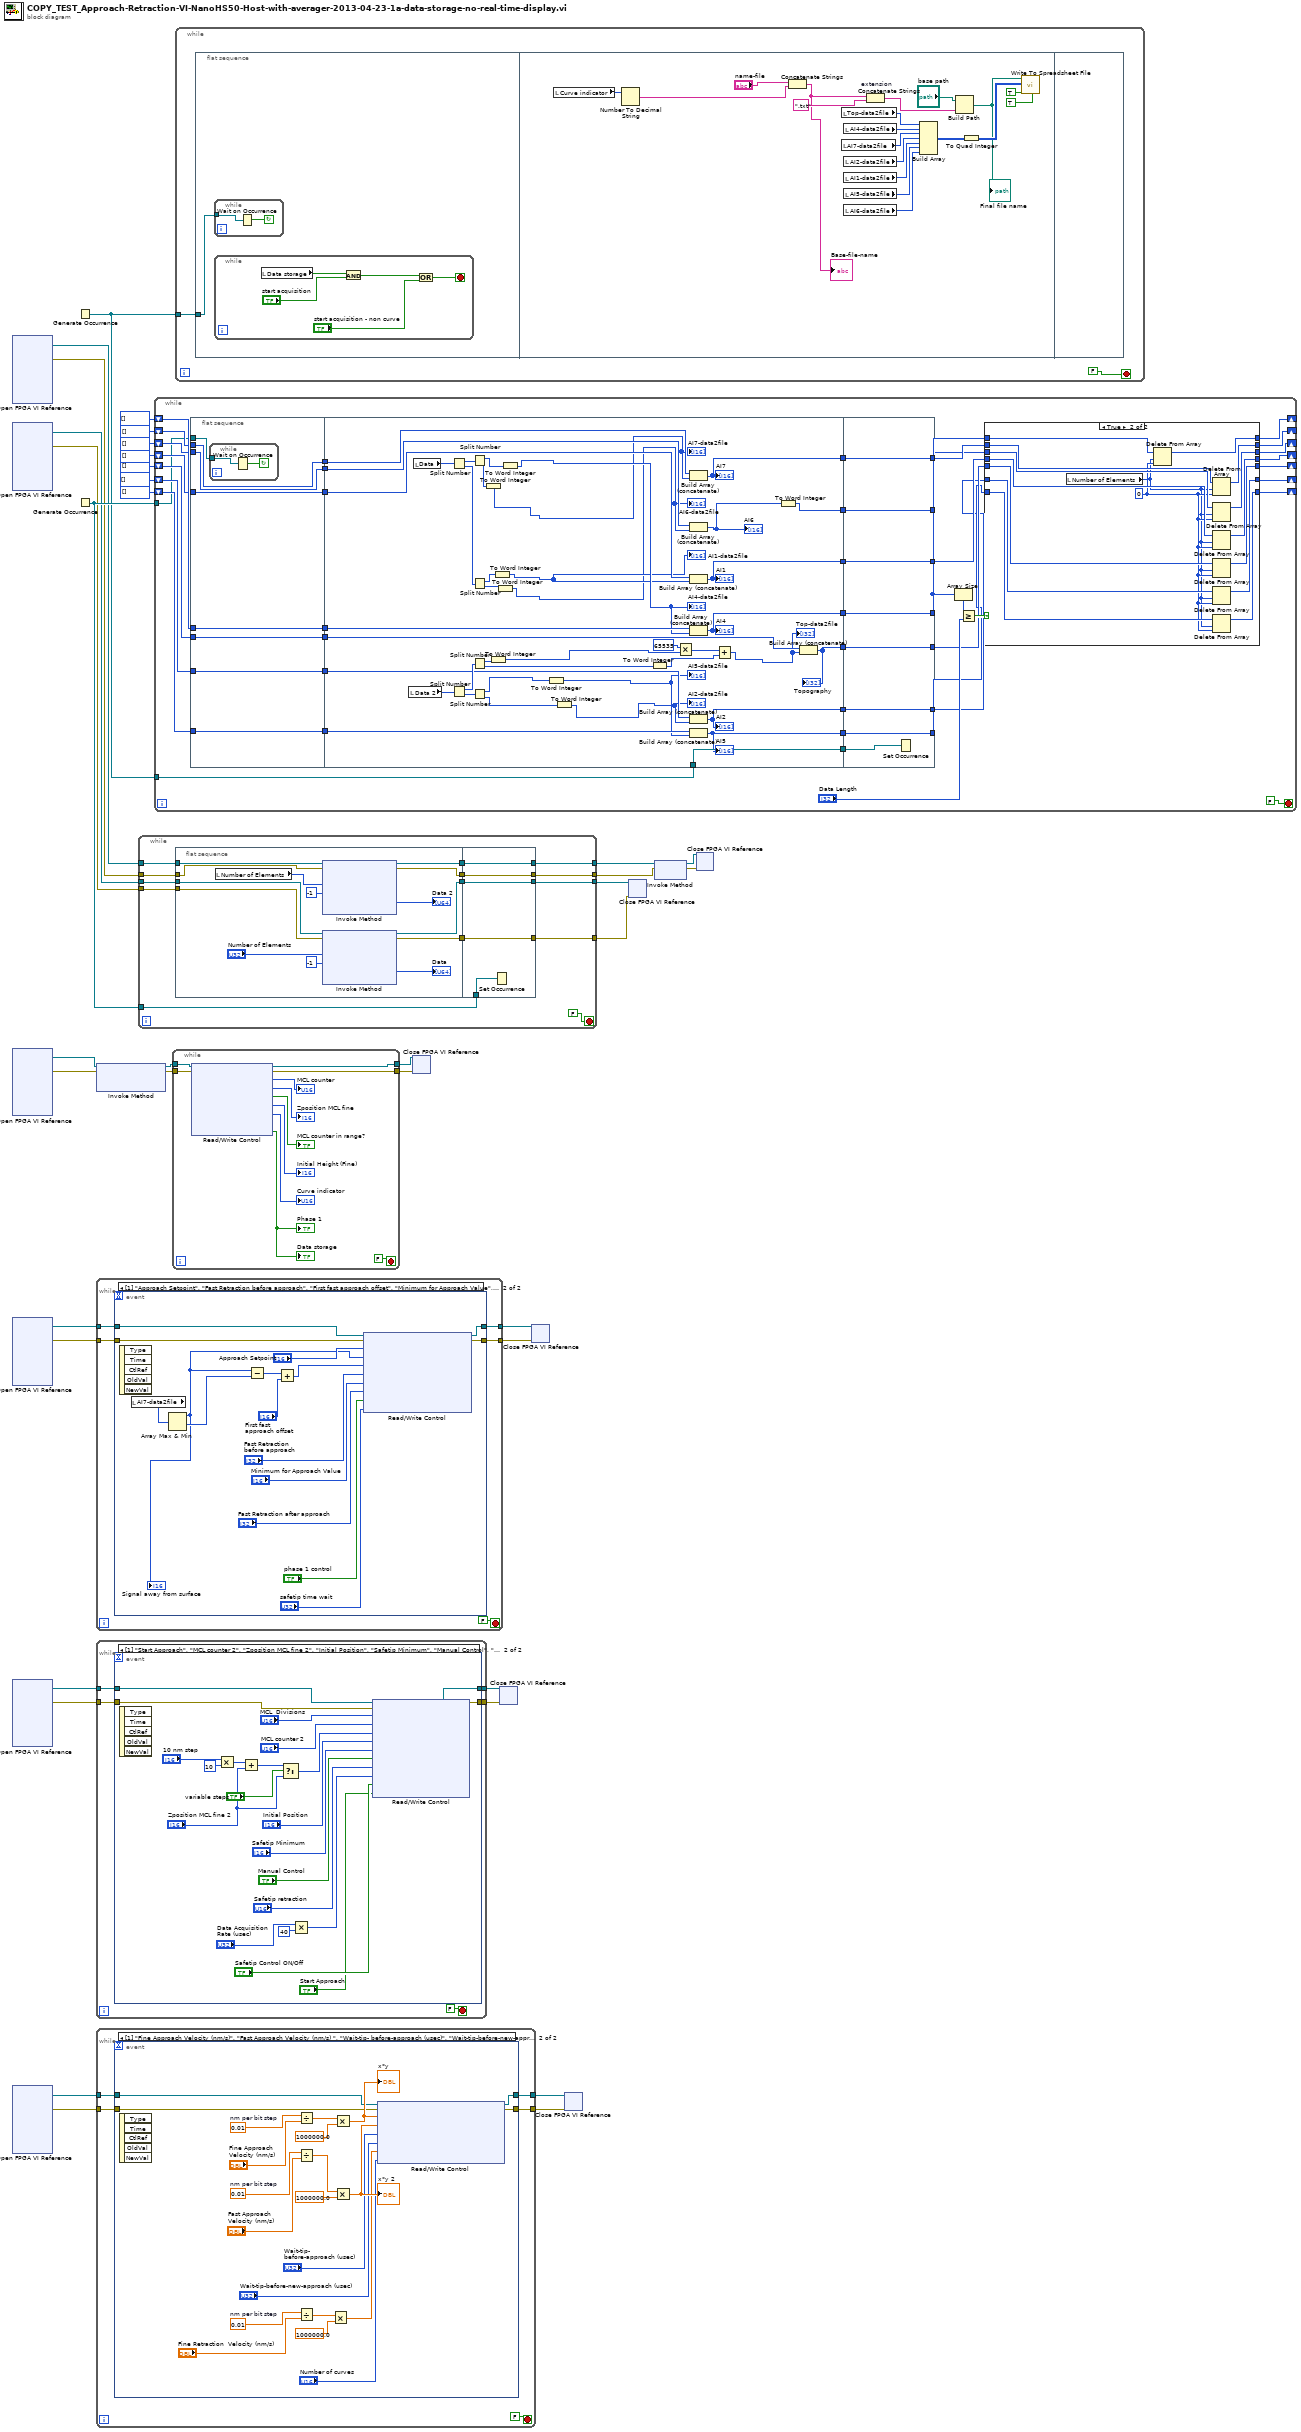
[diagram p0: block diagram]
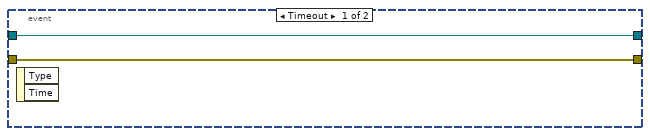
[diagram p2: hidden frame]
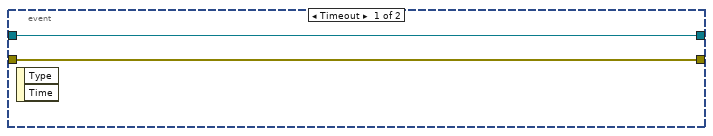
[diagram p3: hidden frame]
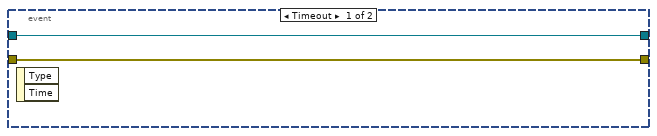
[diagram p4: hidden frame]
diagram:
  n1 = xnode "Open FPGA VI Reference"() -> ("FPGA VI Reference Out"=w22:refnum<k20>, "error out"=w21:errorcluster)  [unwired: 2 in]
  n2 = xnode "Open FPGA VI Reference"() -> ("FPGA VI Reference Out"=w20:refnum<k20>, "error out"=w19:errorcluster)  [unwired: 2 in]
  n3 = xnode "Open FPGA VI Reference"() -> ("FPGA VI Reference Out"=w11:refnum<k20>, "error out"=w9:errorcluster)  [unwired: 2 in]
  n4 = xnode "Open FPGA VI Reference"() -> ("FPGA VI Reference Out"=w26:refnum<k20>, "error out"=w25:errorcluster)  [unwired: 2 in]
  n5 = xnode "Open FPGA VI Reference"() -> ("FPGA VI Reference Out"=w24:refnum<k20>, "error out"=w23:errorcluster)  [unwired: 2 in]
  n6 = xnode "Open FPGA VI Reference"() -> ("FPGA VI Reference Out"=w34:refnum<k20>, "error out"=w33:errorcluster)  [unwired: 2 in]
  n7 = Generate Occurrence() -> (w12:refnum<k4>)
  n8 = Generate Occurrence() -> (w37:refnum<k4>)
  n9 = while {
    tunnel: w26 -> [w42]
    tunnel: w25 -> [w41]
    tunnel: [w39] -> w36
    tunnel: [w38] -> w35
    stop <- FALSE stop-if-true
    n10 = event shown="[1] \"Approach Setpoint\", \"Fast Retraction before approach\", \"First fast approach offset\", \"Minimum for Approach Value\", \"Fast Retraction after approach\", \"Start Approach\", \"phase 1 control\", \"safetip time wait\": Value Change" {
      selector: _ -> [_ _]
      dyn-events: _ -> [_ _]
      timeout: _ -> [_ _]
      tunnel: w42 -> [w44 w60]
      tunnel: w41 -> [w43 w59]
      tunnel: [w44 w54] -> w39
      tunnel: [w43 w53] -> w38
      event Timeout {
        n11 = event-data() -> ()  [unwired: 1 in, 2 out]
      }
      event "Approach Setpoint", "Fast Retraction\nbefore approach", "First fast\napproach offset", "Minimum for Approach Value", "Fast Retraction after approach", "Start Approach", "phase 1 control", "safetip time wait": Value Change {
        n12 = event-data() -> ()  [unwired: 1 in, 5 out]
        n13 = local read "AI7-data2file"() -> (w46:i16[])
        n14 = Array Max & Min(array=w46) -> (max value=w45:i16, min value=w48:i16)  [unwired: 2 out]
        "Signal away from surface" <- w45
        n15 = Subtract(x=w45, y=w48) -> (x-y=w47:i16)
        n16 = Add(x=w47, y="First fast\napproach offset") -> (x+y=w49:i16)
        n17 = xnode "Read/Write Control"("FPGA VI Reference In"=w60, "error in"=w59, "Setpoint Fine"="Approach Setpoint", "TF at infinity"=w45, "Offset for Fast Approach"=w49, "Fast Retraction before approach"="Fast Retraction\nbefore approach", "Minimum for Approach Value"="Minimum for Approach Value", "Fast Retraction After Cycle"="Fast Retraction after approach", "phase 1 control"="phase 1 control", "safetip time wait"="safetip time wait") -> ("FPGA VI Reference Out"=w54:refnum<k20>, "error out"=w53:errorcluster)
      }
    }
  }
  n18 = while {
    tunnel: w23 -> [w65]
    tunnel: w24 -> [w63]
    tunnel: [w62] -> w30
    tunnel: [w61] -> w29
    stop <- FALSE stop-if-true
    n19 = event shown="[1] \"Start Approach\", \"MCL counter 2\", \"Zposition MCL fine 2\", \"Initial Position\", \"Safetip Minimum\", \"Manual Control\", \"Safetip retraction\", \"Safetip Control ON/Off\", \"variable steps\", \"10 nm step\", \"MCL  Divisions\", \"Data Acquisition Rate (usec)\": Value Change" {
      selector: _ -> [_ _]
      dyn-events: _ -> [_ _]
      timeout: _ -> [_ _]
      tunnel: w65 -> [w66 w88]
      tunnel: w63 -> [w67 w89]
      tunnel: [w67 w83] -> w62
      tunnel: [w66 w82] -> w61
      event Timeout {
        n20 = event-data() -> ()  [unwired: 1 in, 2 out]
      }
      event "Start Approach", "MCL counter 2", "Zposition MCL fine 2", "Initial Position", "Safetip Minimum", "Manual Control", "Safetip retraction", "Safetip Control ON/Off", "variable steps", "10 nm step", "MCL  Divisions", "Data Acquisition\nRate (usec)": Value Change {
        n21 = event-data() -> ()  [unwired: 1 in, 5 out]
        n22 = Multiply(x="10 nm step", y=i16 10) -> (x*y=w75:i16)
        n23 = Add(x=w75, y="Zposition MCL fine 2") -> (x+y=w73:i16)
        n24 = Select(t=w73, s="variable steps", f="Zposition MCL fine 2") -> (s? t:f=w78:i16)
        n25 = Multiply(x="Data Acquisition\nRate (usec)", y=u32 40) -> (x*y=w70:u32)
        n26 = xnode "Read/Write Control"("FPGA VI Reference In"=w89, "error in"=w88, "MCL Divisions"="MCL  Divisions", "MCL counter 2"="MCL counter 2", "Zposition MCL fine 2"=w78, "Initial Position"="Initial Position", "Safetip Minimum"="Safetip Minimum", "Manual Control"="Manual Control", "Safetip retraction"="Safetip retraction", "Data Acquisition Rate (usec)"=w70, "Safetip Control ON/Off"="Safetip Control ON/Off", "Start Approach"="Start Approach") -> ("FPGA VI Reference Out"=w83:refnum<k20>, "error out"=w82:errorcluster)
      }
    }
  }
  n27 = while {
    tunnel: w34 -> [w94]
    tunnel: w33 -> [w93]
    tunnel: [w92] -> w32
    tunnel: [w91] -> w31
    stop <- FALSE stop-if-true
    n28 = event shown="[1] \"Fine Approach Velocity (nm/s)\", \"Fast Approach Velocity (nm/s) \", \"Wait-tip- before-approach (usec)\", \"Wait-tip-before-new-approach (usec)\", \"Fine Retraction  Velocity (nm/s) \", \"Number of curves\": Value Change" {
      selector: _ -> [_ _]
      dyn-events: _ -> [_ _]
      timeout: _ -> [_ _]
      tunnel: w94 -> [w96 w100]
      tunnel: w93 -> [w95 w99]
      tunnel: [w96 w98] -> w92
      tunnel: [w95 w97] -> w91
      event Timeout {
        n29 = event-data() -> ()  [unwired: 1 in, 2 out]
      }
      event "Fine Approach\nVelocity (nm/s)", "Fast Approach\nVelocity (nm/s)", "Wait-tip-\nbefore-approach (usec)", "Wait-tip-before-new-approach (usec)", "Fine Retraction  Velocity (nm/s)", "Number of curves": Value Change {
        w106 = 0.01  # nm per bit step
        w111 = 0.01  # nm per bit step
        w117 = 0.01  # nm per bit step
        n30 = event-data() -> ()  [unwired: 1 in, 5 out]
        n31 = Divide(x=w117, y="Fine Approach\nVelocity (nm/s)") -> (x/y=w116:dbl)
        n32 = Divide(x=w111, y="Fast Approach\nVelocity (nm/s)") -> (x/y=w112:dbl)
        n33 = Divide(x=w106, y="Fine Retraction  Velocity (nm/s)") -> (x/y=w104:dbl)
        n34 = Multiply(x=w104, y=1000000.0) -> (x*y=w102:dbl)
        n35 = Multiply(x=w116, y=1000000.0) -> (x*y=w114:dbl)
        "x*y" <- w114
        n36 = Multiply(x=w112, y=1000000.0) -> (x*y=w109:dbl)
        "x*y 2" <- w109
        n37 = xnode "Read/Write Control"("FPGA VI Reference In"=w100, "error in"=w99, "Fine Approach (usec)"=w114, "Fast Approach (usec)"=w109, "Wait-tip-before-approach"="Wait-tip-\nbefore-approach (usec)", "Wait-tip-before-new-approach (usec)"="Wait-tip-before-new-approach (usec)", "Fine Retraction (usec)"=w102, "Number of curves"="Number of curves") -> ("FPGA VI Reference Out"=w98:refnum<k20>, "error out"=w97:errorcluster)
      }
    }
  }
  n38 = xnode "Invoke Method"("FPGA VI Reference In"=w11, "error in"=w9) -> ("FPGA VI Reference Out"=w10:refnum<k20>, "error out"=w8:errorcluster)  [unwired: 1 in]
  n39 = while {
    tunnel: w37 -> [w128]
    tunnel: w22 -> [w127]
    tunnel: w21 -> [w126]
    tunnel: w20 -> [w125]
    tunnel: w19 -> [w124]
    tunnel: [w123] -> w14
    tunnel: [w122] -> w16
    tunnel: [w121] -> w17
    tunnel: [w120] -> w18
    stop <- FALSE stop-if-true
    n40 = flat-sequence {
      tunnel: [w146] -> w132
      tunnel: [w145] -> w131
      tunnel: [w144] -> w130
      tunnel: [w143] -> w129
      tunnel: w127 -> [w136]
      tunnel: w126 -> [w135]
      tunnel: w125 -> [w134]
      tunnel: w124 -> [w133]
      tunnel: [w148] -> w122
      tunnel: [w149] -> w123
      tunnel: [w150] -> w120
      tunnel: [w151] -> w121
      tunnel: w132 -> [w151]
      tunnel: w131 -> [w150]
      tunnel: w130 -> [w149]
      tunnel: w129 -> [w148]
      tunnel: w128 -> [w147]
      frame #0 {
        n41 = local read "Number of Elements"() -> (w142:u32)
        n42 = xnode "Invoke Method"("FPGA VI Reference In"=w136, "error in"=w135, "Number of Elements"=w142, "Timeout (ms)"=-1) -> ("FPGA VI Reference Out"=w144:refnum<k20>, "error out"=w143:errorcluster, "Data"=→"Data 2":i16[])  [unwired: 1 out]
        n43 = xnode "Invoke Method"("FPGA VI Reference In"=w134, "error in"=w133, "Number of Elements"="Number of Elements", "Timeout (ms)"=-1) -> ("FPGA VI Reference Out"=w146:refnum<k20>, "error out"=w145:errorcluster, "Data"=→"Data":u64[])  [unwired: 1 out]
      }
      frame #1 {
        n44 = Set Occurrence(w147) -> ()
      }
    }
  }
  n45 = while {
    shift-right: [w173] -> _
    shift-left: i16[] [] -> [w193]
    shift-right: [w161] -> _
    shift-left: i16[] [] -> [w192]
    shift-right: [w163] -> _
    shift-left: i16[] [] -> [w191]
    shift-right: [w162] -> _
    shift-left: i16[] [] -> [w190]
    shift-right: [w166] -> _
    shift-left: i32[] [] -> [w189]
    shift-right: [w164] -> _
    shift-left: i16[] [] -> [w188]
    shift-right: [w165] -> _
    shift-left: i16[] [] -> [w187]
    tunnel: w37 -> [w178]
    tunnel: w12 -> [w152]
    stop <- FALSE stop-if-true
    n46 = flat-sequence {
      tunnel: w187 -> [w218]
      tunnel: w188 -> [w219]
      tunnel: w189 -> [w220]
      tunnel: w190 -> [w221]
      tunnel: w191 -> [w222]
      tunnel: w192 -> [w223]
      tunnel: w193 -> [w224]
      tunnel: [w224] -> w185
      tunnel: [w223] -> w184
      tunnel: [w222] -> w183
      tunnel: [w221] -> w182
      tunnel: [w220] -> w181
      tunnel: [w219] -> w180
      tunnel: [w218] -> w179
      tunnel: w178 -> [w217]
      tunnel: w185 -> [w261]
      tunnel: w184 -> [w260]
      tunnel: w183 -> [w255]
      tunnel: w182 -> [w254]
      tunnel: w181 -> [w258]
      tunnel: w180 -> [w252]
      tunnel: w179 -> [w253]
      tunnel: [w251] -> w160
      tunnel: [w249] -> w159
      tunnel: [w228] -> w158
      tunnel: [w259] -> w157
      tunnel: [w245] -> w156
      tunnel: [w244] -> w155
      tunnel: [w250] -> w154
      tunnel: [w246] -> w153
      tunnel: w152 -> [w246]
      tunnel: [w269] -> w172
      tunnel: [w270] -> w168
      tunnel: [w271] -> w167
      tunnel: [w272] -> w169
      tunnel: [w273] -> w171
      tunnel: [w274] -> w170
      tunnel: [w275] -> w174
      tunnel: w160 -> [w275]
      tunnel: w159 -> [w274]
      tunnel: w158 -> [w273]
      tunnel: w157 -> [w272]
      tunnel: w156 -> [w271]
      tunnel: w155 -> [w270]
      tunnel: w154 -> [w269]
      tunnel: w153 -> [w268]
      frame #0 {
        n47 = while {
          tunnel: w217 -> [w225]
          stop <- w226 continue-if-true
          n48 = Wait on Occurrence(2:w225) -> (0:w226:bool)  [unwired: 2 in]
        }
      }
      frame #1 {
        n49 = local read "Data 2"() -> (w262:u64[])
        n50 = local read "Data"() -> (w265:u64[])
        n51 = Split Number(x=w265) -> (hi(x)=w267:u32[], lo(x)=w266:u32[])
        n52 = Split Number(x=w262) -> (hi(x)=w264:u32[], lo(x)=w263:u32[])
        n53 = Split Number(x=w267) -> (hi(x)=w241:u16[], lo(x)=w240:u16[])
        n54 = Split Number(x=w266) -> (hi(x)=w243:u16[], lo(x)=w242:u16[])
        n55 = Split Number(x=w264) -> (hi(x)=w239:u16[], lo(x)=w248:u16[])
        n56 = Split Number(x=w263) -> (hi(x)=w237:u16[], lo(x)=w236:u16[])
        n57 = To Word Integer(number=w240) -> (16bit integer=w234:i16[])
        "AI7-data2file" <- w234
        n58 = To Word Integer(number=w239) -> (16bit integer=w238:i16[])
        n59 = To Word Integer(number=w243) -> (16bit integer=w233:i16[])
        "AI1-data2file" <- w233
        n60 = To Word Integer(number=w242) -> (16bit integer=w232:i16[])
        "AI6-data2file" <- w232
        n61 = To Word Integer(number=w241) -> (16bit integer=w235:i16[])
        "AI4-data2file" <- w235
        n62 = To Word Integer(number=w237) -> (16bit integer=w231:i16[])
        "AI5-data2file" <- w231
        n63 = To Word Integer(number=w236) -> (16bit integer=w230:i16[])
        "AI2-data2file" <- w230
        n64 = To Word Integer(number=w248) -> (16bit integer=w247:i16[])
        n65 = Multiply(x=65535, y=w238) -> (x*y=w256:i32[])
        n66 = Build Array (concatenate)(w260, w234) -> (w250:i16[])
        "AI7" <- w250
        n67 = Build Array (concatenate)(w255, w232) -> (w229:i16[])
        "AI6" <- w229
        n68 = Build Array (concatenate)(w254, w233) -> (w249:i16[])
        "AI1" <- w249
        n69 = Build Array (concatenate)(w261, w235) -> (w251:i16[])
        "AI4" <- w251
        n70 = Build Array (concatenate)(w252, w230) -> (w245:i16[])
        "AI2" <- w245
        n71 = Build Array (concatenate)(w253, w231) -> (w244:i16[])
        "AI5" <- w244
        n72 = Add(x=w256, y=w247) -> (x+y=w227:i32[])
        "Top-data2file" <- w227
        n73 = To Word Integer(number=w229) -> (16bit integer=w228:i16[])
        n74 = Build Array (concatenate)(w258, w227) -> (w259:i32[])
        "Topography" <- w259
      }
      frame #2 {
        n75 = Set Occurrence(w268) -> ()
      }
    }
    n76 = Array Size(array=w174) -> (size(s)=w177:i32)
    n77 = Greater Or Equal?(x=w177, y="Data Length") -> (x >= y?=w175:bool)
    n78 = case shown="True" w175 {
      tunnel: w174 -> [w200 w216]
      tunnel: [w200 w215] -> w173
      tunnel: w172 -> [w199 w214]
      tunnel: [w199 w213] -> w161
      tunnel: w171 -> [w198 w208]
      tunnel: w170 -> [w197 w209]
      tunnel: w169 -> [w196 w210]
      tunnel: w168 -> [w195 w211]
      tunnel: w167 -> [w194 w212]
      tunnel: [w198 w206] -> w163
      tunnel: [w197 w205] -> w162
      tunnel: [w196 w204] -> w166
      tunnel: [w195 w203] -> w165
      tunnel: [w194 w202] -> w164
      frame False {
      }
      frame True {
        w207 = 0 ("index")
        n79 = local read "Number of Elements"() -> (w201:u32)
        n80 = Delete From Array "Delete From Array"(array=w216, length=w201, index=w207) -> (array with subset deleted=w215:i16[])  [unwired: 1 out]
        n81 = Delete From Array(array=w214, length=w201, index=w207) -> (array with subset deleted=w213:i16[])  [unwired: 1 out]
        n82 = Delete From Array(array=w208, length=w201, index=w207) -> (array with subset deleted=w206:i16[])  [unwired: 1 out]
        n83 = Delete From Array(array=w209, length=w201, index=w207) -> (array with subset deleted=w205:i16[])  [unwired: 1 out]
        n84 = Delete From Array(array=w210, length=w201, index=w207) -> (array with subset deleted=w204:i32[])  [unwired: 1 out]
        n85 = Delete From Array(array=w212, length=w201, index=w207) -> (array with subset deleted=w202:i16[])  [unwired: 1 out]
        n86 = Delete From Array(array=w211, length=w201, index=w207) -> (array with subset deleted=w203:i16[])  [unwired: 1 out]
      }
    }
  }
  n87 = while {
    tunnel: w10 -> [w286]
    tunnel: [w285] -> w28
    tunnel: [w284] -> w27
    tunnel: w8 -> [w283]
    stop <- FALSE stop-if-true
    n88 = xnode "Read/Write Control"("FPGA VI Reference In"=w286, "error in"=w283) -> ("FPGA VI Reference Out"=w285:refnum<k20>, "error out"=w284:errorcluster, "MCL counter"=→"MCL counter":u16, "Zposition MCL fine"=→"Zposition MCL fine":i16, "MCL counter in range?"=→"MCL counter in range?":bool, "Initial Height (Fine)"=→"Initial Height (Fine)":i16, "Curve indicator"=→"Curve indicator":u16, "Data storage"=→"Phase 1" →"Data storage":bool)  [unwired: 1 out]
  }
  n89 = while {
    tunnel: w12 -> [w288]
    stop <- FALSE stop-if-true
    n90 = flat-sequence {
      tunnel: w288 -> [w289]
      frame #0 {
        n91 = while {
          tunnel: w289 -> [w290]
          stop <- w291 continue-if-true
          n92 = Wait on Occurrence(2:w290) -> (0:w291:bool)  [unwired: 2 in]
        }
        n93 = while {
          stop <- w292 stop-if-true
          n94 = local read "Data storage"() -> (w295:bool)
          n95 = And(x=w295, y="start acquisition") -> (x .and. y?=w296:bool)
          n96 = Or(x=w296, y="start acquisition - non curve") -> (x .or. y?=w292:bool)
        }
      }
      frame #1 {
        n97 = local read "Curve indicator"() -> (w300:u16)
        n98 = Number To Decimal String(number=w300) -> (decimal integer string=w303:string)  [unwired: 1 in]
        n99 = Concatenate Strings "Concatenate Strings"("name-file", w303) -> (w298:string)
        "Base-file-name" <- w298
        n100 = local read "Top-data2file"() -> (w305:i32[])
        n101 = local read "AI7-data2file"() -> (w314:i16[])
        n102 = local read "AI4-data2file"() -> (w315:i16[])
        n103 = local read "AI2-data2file"() -> (w312:i16[])
        n104 = local read "AI1-data2file"() -> (w311:i16[])
        n105 = local read "AI5-data2file"() -> (w310:i16[])
        n106 = local read "AI6-data2file"() -> (w309:i16[])
        n107 = Concatenate Strings "extension"(w298, ".txt" ("string")) -> (w297:string)
        n108 = Build Array(w305, w315, w314, w312, w311, w310, w309) -> (w307:i32[][])
        n109 = Build Path(base path="base path", name or relative path=w297) -> (appended path=w301:path)
        "Final file name" <- w301
        n110 = To Quad Integer(1:w307) -> (0:w306:i64[][])
        n111 = call-poly <vilib>:"Write To Spreadsheet File.vi"("transpose? (no:F)"=TRUE, "append to file? (new file:F)"=TRUE, "2D data"=w306, "file path (dialog if empty)"=w301) -> ()  [unwired: 4 in, 1 out]
      }
      frame #2 {
      }
    }
  }
  n112 = xnode "Close FPGA VI Reference"("FPGA VI Reference In"=w28, "error in"=w27) -> ()  [unwired: 1 out]
  n113 = xnode "Close FPGA VI Reference"("FPGA VI Reference In"=w30, "error in"=w29) -> ()  [unwired: 1 out]
  n114 = xnode "Close FPGA VI Reference"("FPGA VI Reference In"=w36, "error in"=w35) -> ()  [unwired: 1 out]
  n115 = xnode "Close FPGA VI Reference"("FPGA VI Reference In"=w32, "error in"=w31) -> ()  [unwired: 1 out]
  n116 = xnode "Close FPGA VI Reference"("FPGA VI Reference In"=w17, "error in"=w18) -> ()  [unwired: 1 out]
  n117 = xnode "Invoke Method"("FPGA VI Reference In"=w14, "error in"=w16) -> ("FPGA VI Reference Out"=w13:refnum<k20>, "error out"=w15:errorcluster)
  n118 = xnode "Close FPGA VI Reference"("FPGA VI Reference In"=w13, "error in"=w15) -> ()  [unwired: 1 out]
